vi "main.vi"() -> ()   [LabVIEW 2025]
doc: "This VI illustrates how to play a sound file continuously, reading the sound file in pieces, and playing each piece at a time."
uses:
  <vilib>/sound2/lvsound2.llb/Sampling Mode.ctl
  <vilib>/sound2/lvsound2.llb/Sound File Info (path).vi
  <vilib>/sound2/lvsound2.llb/Sound File Read Open.vi
  <vilib>/sound2/lvsound2.llb/Sound File Read (DBL).vi
  <vilib>/express/express analysis/Spectral/Block/exnSpectralBlock spectral measurements RMS poly.vi
  <vilib>/express/express analysis/Spectral/Block/exnSpectralBlock spectral measurements RMS array WFM.vi
  <vilib>/sound2/lvsound2.llb/Sound Output Write (DBL).vi
  <vilib>/express/express analysis/Spectral/XNode/ExpressSpectralMeasurementsBlockNode.xnode
panel:
  out "Output Spectrum":cluster{"f0":dbl, "df":dbl, "magnitude":dbl[]}[](graph)
  out "Input Spectrum":cluster{"f0":dbl, "df":dbl, "magnitude":dbl[]}[](graph)
  out "Filtered Current Data":waveform(dbl)[](graph)
  in  "High 2400+ Hz (dB)":dbl(slide)=10.0 scale=-10.0..10.0 scale format="%#_20g"
  in  "Medium 200-2400 Hz (dB)":dbl(slide)=-4.261954261954262 scale=-10.0..10.0 scale format="%#_20g"
  in  "Low 0-200 Hz (dB)":dbl(slide)=4.012474012474014 scale=-10.0..10.0 scale format="%#_20g"
  out "Current Data":waveform(dbl)[](graph)
  out "Current Iteration":i32
  in  "Stop":bool
  in  "Number of Samples/Iteration":i32=2500
  in  "Device ID":u32
  # "Overview: Demonstrates the use of the Sound VIs to play a sound file continuously, reading the sound file in pieces, and playing each piece one at a time.\nInstructions:\n1. Specify the Device ID and the Number of Samples/Iteration.\n2. Run the VI."
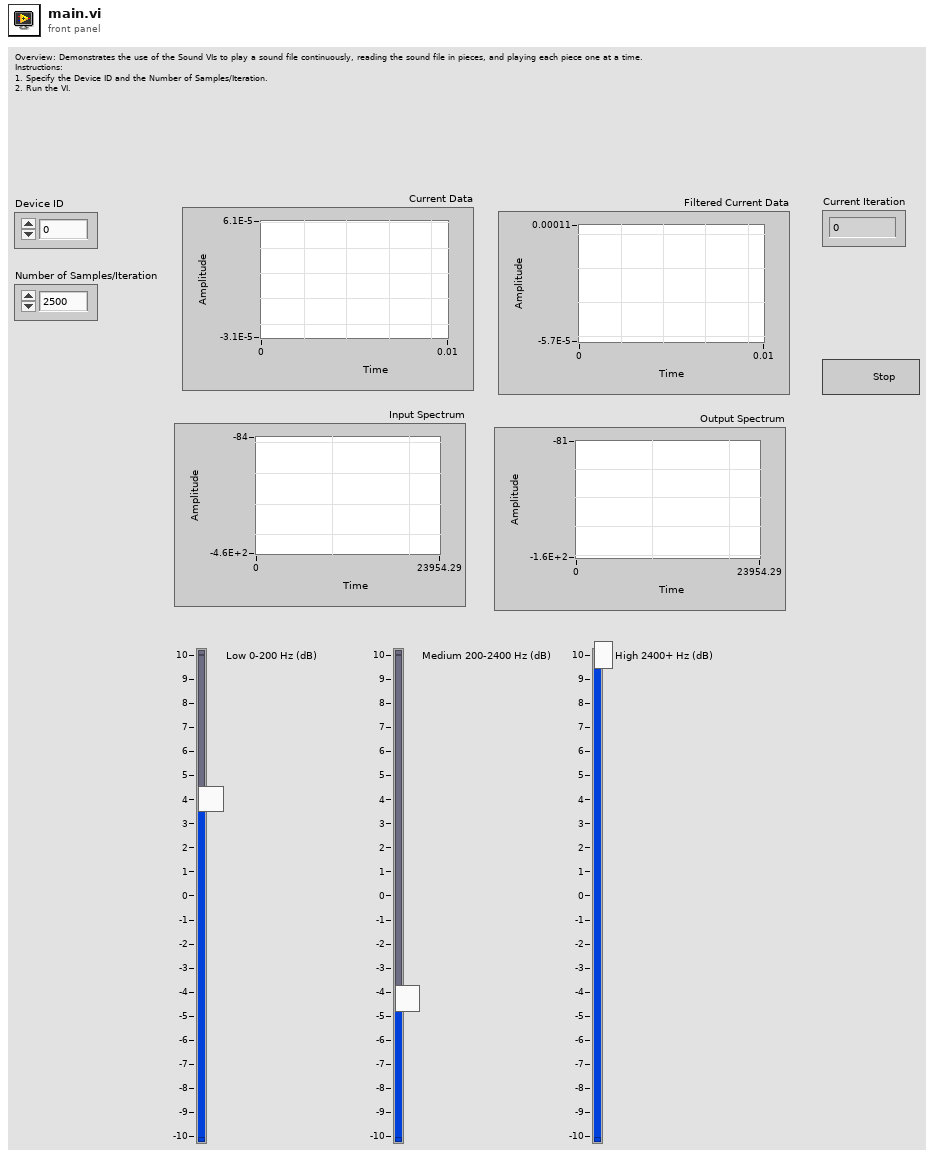
[diagram p1: front panel]
types:
  T1 = typedef "Sampling Mode.ctl" = i32
  T2 = typedef "Sound Data Format.ctl" = cluster{"sample rate (S/s)":dbl, "number of channels":i32, "bits per sample":i32}
  T3 = typedef "Sound File Refnum.ctl" = refnum<file>
  T4 = typedef "Sound Output Task ID.ctl" = u32
  T5 = cluster{"averaging mode":u16, "weighting mode":u16, "number of averages":u32}
  T6 = cluster{"dB On (F)":bool, "unwrap phase (F)":bool, "convert to degree (F)":bool}
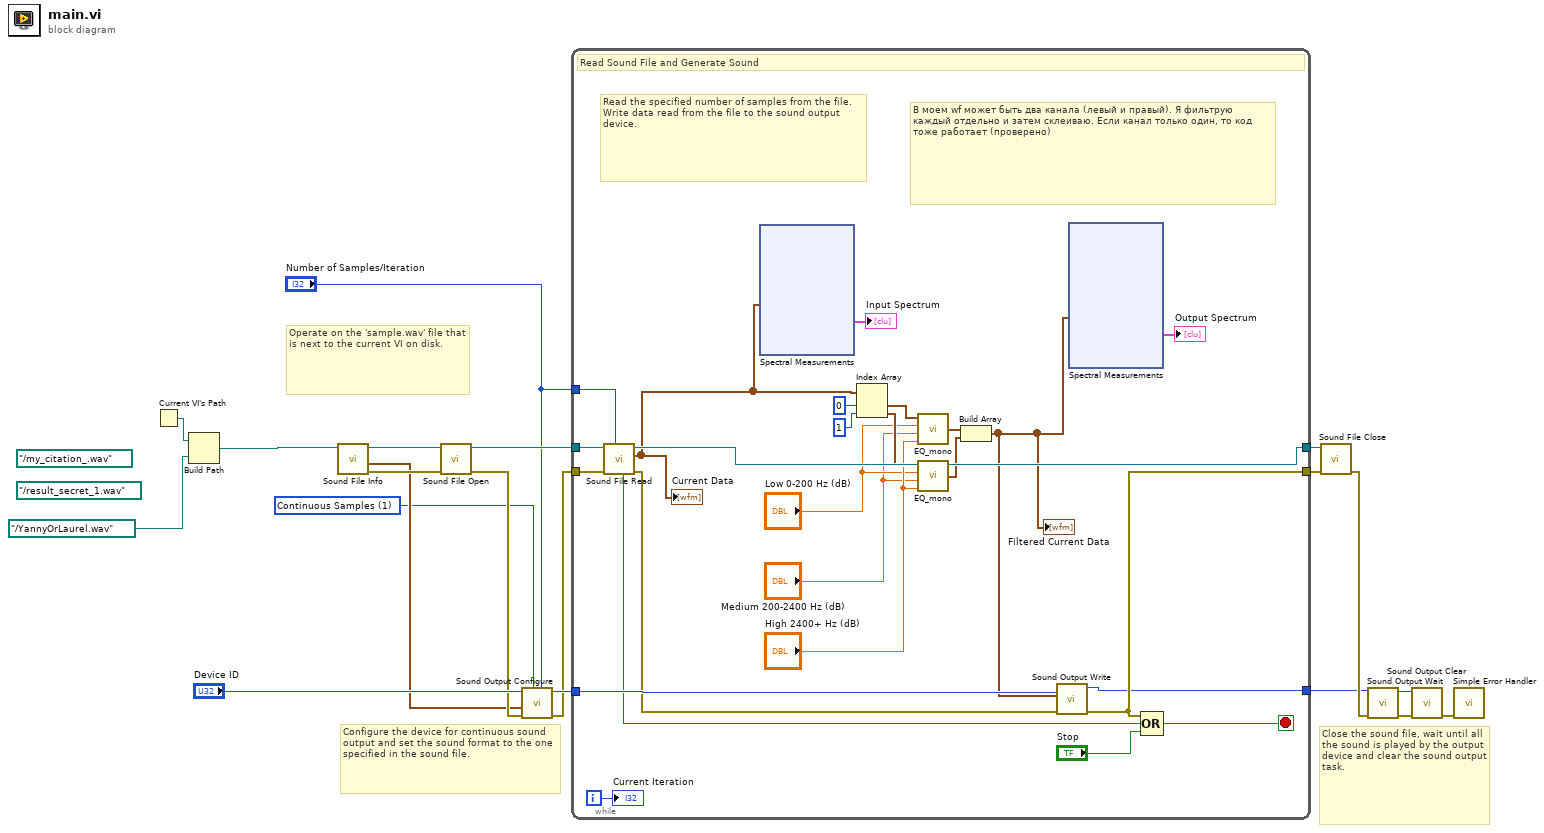
[diagram p0: block diagram]
diagram:
  (unwired) path "../result_secret_1.wav" ("Sound File Path")
  (unwired) path "../my_citation_.wav" ("Sound File Path")
  w6 = T1 1 items=["Finite Samples", "Continuous Samples"] ("sample mode")
  # "Operate on the 'sample.wav' file that is next to the current VI on disk."
  # "Close the sound file, wait until all the sound is played by the output device and clear the sound output task."
  # "Configure the device for continuous sound output and set the sound format to the one specified in the sound file."
  n1 = Current VI's Path() -> (path=w3:path)
  n2 = Build Path(base path=w3, name or relative path=path "../YannyOrLaurel.wav" ("Sound File Path")) -> (appended path=w4:path)
  n3 = call-poly <vilib>:"Sound File Info.vi"("path"=w4) -> ("error out"=w15:errorcluster, "sound format"=w8:T2, "path out"=w9:path)  [unwired: 7 in, 1 out]
  n4 = call-poly <vilib>:"Sound File Open.vi"("error in (no error)"=w15, "path"=w9) -> ("error out"=w14:errorcluster, "sound file refnum"=w16:T3)  [unwired: 8 in]
  n5 = call <vilib>:"Sound Output Configure.vi"("number of samples/ch"="Number of Samples/Iteration", "sample mode"=w6, "error in (no error)"=w14, "sound format"=w8, "device ID"="Device ID") -> ("error out"=w13:errorcluster, "task ID"=w20:T4)  [unwired: 5 in]
  n6 = while {
    tunnel: "Number of Samples/Iteration" -> [w36]
    tunnel: w16 -> [w44]
    tunnel: [w42] -> w18
    tunnel: w13 -> [w45]
    tunnel: [w35] -> w17
    tunnel: w20 -> [w41]
    tunnel: [w34] -> w2
    i -> [w43]
    stop <- w37 stop-if-true
    # "В моем wf может быть два канала (левый и правый). Я фильтрую каждый отдельно и затем склеиваю. Если канал только один, то код тоже работает (проверено)"
    # "Read the specified number of samples from the file. Write data read from the file to the sound output device."
    # "Read Sound File and Generate Sound"
    n7 = call-poly <vilib>:"Sound File Read.vi"("number of samples/ch (-1: all)"=w36, "error in (no error)"=w45, "sound file refnum"=w44) -> ("error out"=w40:errorcluster, "data"=w26:waveform(dbl)[], "sound file refnum out"=w42:T3, "end of file?"=w38:bool)  [unwired: 4 in, 1 out]
    "Current Data" <- w26
    n8 = xnode "Spectral Measurements"("Signals"=w26) -> ("FFT - (RMS)"=→"Input Spectrum":cluster{"f0":dbl, "df":dbl, "magnitude":dbl[]}[])  [unwired: 1 in, 2 out]
    n9 = Index Array(array=w26, index #1=0 ("index"), index #2=1 ("index")) -> (element #1=w31:waveform(dbl), element #2=w30:waveform(dbl))
    n10 = call "EQ_mono.vi"("High 2400+ Hz (dB)"="High 2400+ Hz (dB)", "Medium 200-2400 Hz (dB)"="Medium 200-2400 Hz (dB)", "Low 0-200 Hz (dB)"="Low 0-200 Hz (dB)", "Audio in"=w31) -> ("output waveform"=w28:waveform(dbl))
    n11 = call "EQ_mono.vi"("High 2400+ Hz (dB)"="High 2400+ Hz (dB)", "Medium 200-2400 Hz (dB)"="Medium 200-2400 Hz (dB)", "Low 0-200 Hz (dB)"="Low 0-200 Hz (dB)", "Audio in"=w30) -> ("output waveform"=w27:waveform(dbl))
    n12 = Build Array(w28, w27) -> (w23:waveform(dbl)[])
    "Filtered Current Data" <- w23
    n13 = call-poly <vilib>:"Sound Output Write.vi"("error in (no error)"=w40, "data"=w23, "task ID"=w41) -> ("error out"=w35:errorcluster, "task ID out"=w34:T4)  [unwired: 7 in]
    n14 = xnode "Spectral Measurements"("Signals"=w23) -> ("FFT - (RMS)"=→"Output Spectrum":cluster{"f0":dbl, "df":dbl, "magnitude":dbl[]}[])  [unwired: 1 in, 2 out]
    n15 = Compound Arithmetic op=OR(w35, w38, "Stop") -> (w37:bool)
    "Current Iteration" <- w43
  }
  n16 = call <vilib>:"Sound File Close.vi"("error in (no error)"=w17, "sound file refnum"=w18) -> ("error out"=w11:errorcluster)  [unwired: 9 in]
  n17 = call <vilib>:"Sound Output Wait.vi"("error in (no error)"=w11, "task ID"=w2) -> ("error out"=w10:errorcluster, "task ID out"=w12:T4)  [unwired: 8 in]
  n18 = call <vilib>:"Sound Output Clear.vi"("error in (no error)"=w10, "task ID"=w12) -> ("error out"=w5:errorcluster)  [unwired: 9 in]
  n19 = call <vilib>:"Simple Error Handler.vi"("error in (no error)"=w5) -> ()  [unwired: 4 in, 5 out]
